vi "Demapper.vi"(8 "OFDM symbol index":u16, 9 "configuration":T4={"primary channel selector"=0.0, "last OFDM symbol index"=0, "switch format detection states"=TRUE, "format"=enum."NON_HT_OFDM", "bandwidth"=enum."20MHz"}, 10 "input valid":bool=TRUE, 11 "subcarrier channels":T1) -> (0 "subcarrier index":fxp<+/-,9,9>, 1 "subcarrier timing":T3={"subcarrier index"=0, "OFDM symbol index"=0, "frequency offset index"=0.0, "OFDM symbol start"=TRUE, "valid"=TRUE}, 2 "field map":T2, 3 "subcarrier channels out":T1)   [LabVIEW 2020]
uses:
  FPGA Bitfiles/Configuration Control.ctl
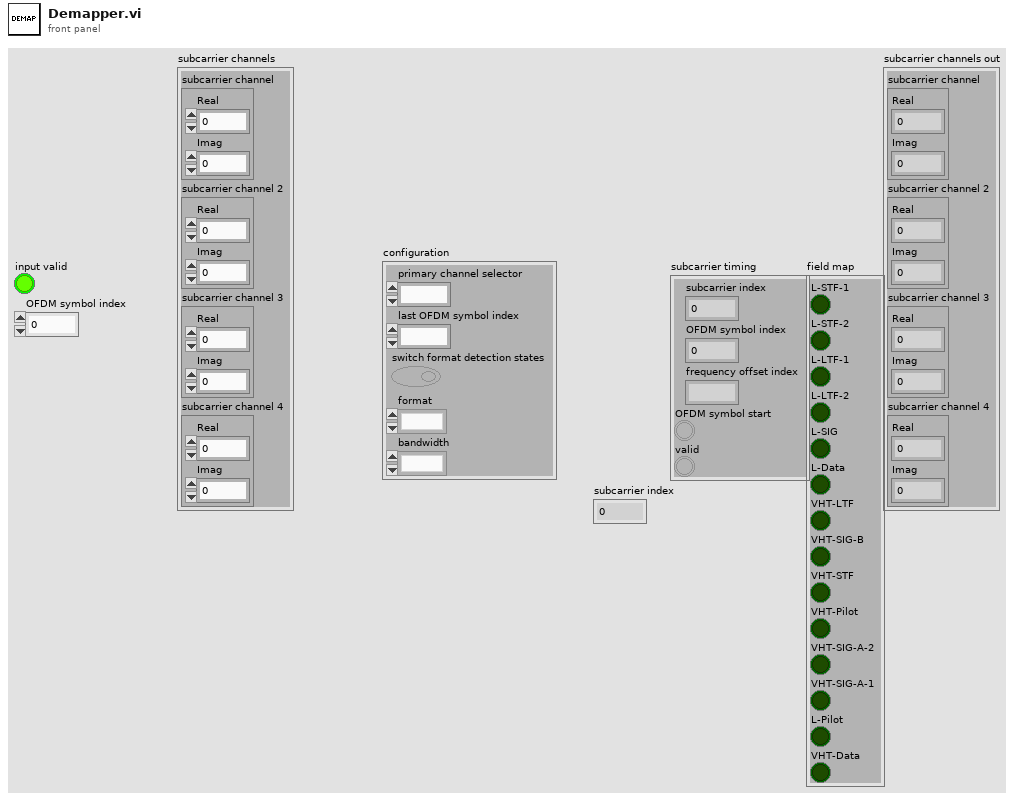
[diagram p1: front panel]
types:
  T1 = cluster{"subcarrier channel":cluster{"Real":fxp<+/-,25,4>, "Imag":fxp<+/-,25,4>}, "subcarrier channel 2":cluster{"Real":fxp<+/-,25,4>, "Imag":fxp<+/-,25,4>}, "subcarrier channel 3":cluster{"Real":fxp<+/-,25,4>, "Imag":fxp<+/-,25,4>}, "subcarrier channel 4":cluster{"Real":fxp<+/-,25,4>, "Imag":fxp<+/-,25,4>}}
  T2 = cluster{"L-STF-1":bool, "L-STF-2":bool, "L-LTF-1":bool, "L-LTF-2":bool, "L-SIG":bool, "L-Data":bool, "VHT-LTF":bool, "VHT-SIG-B":bool, "VHT-STF":bool, "VHT-Pilot":bool, "VHT-SIG-A-2":bool, "VHT-SIG-A-1":bool, "L-Pilot":bool, "VHT-Data":bool}
  T3 = cluster{"subcarrier index":u8, "OFDM symbol index":u16, "frequency offset index":fxp<+/-,9,9>, "OFDM symbol start":bool, "valid":bool}
  T4 = typedef "Configuration Control.ctl" = cluster{"primary channel selector":fxp<+,2,0>, "last OFDM symbol index":u16, "switch format detection states":bool, "format":enum16{"NON_HT_OFDM", "VHT", "NON_HT_DUP_OFDM"}, "bandwidth":enum16{"20MHz", "40MHz", "80MHz"}}
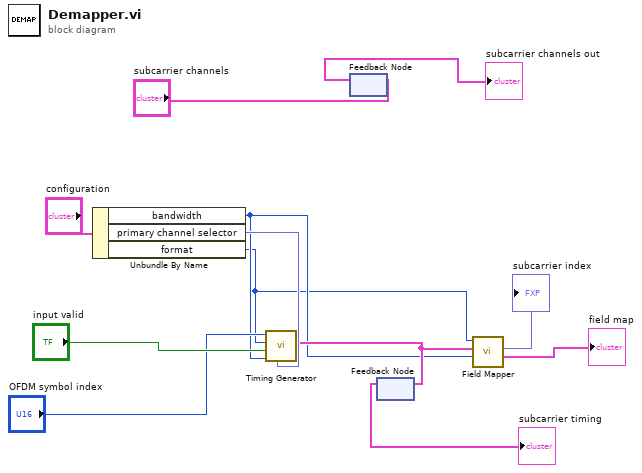
[diagram p0: block diagram]
diagram:
  n1 = Unbundle By Name("configuration") -> ("bandwidth"=w6:enum16{"20MHz", "40MHz", "80MHz"}, "primary channel selector"=w9:fxp<+,2,0>, "format"=w5:enum16{"NON_HT_OFDM", "VHT", "NON_HT_DUP_OFDM"})
  n2 = call "Timing Generator.vi"("primary channel selector"=w9, "bandwidth"=w6, "enable subcarrier counter"="input valid", "format"=w5, "OFDM symbol index"="OFDM symbol index") -> ("Cluster timing"=w7:T3)  [unwired: 6 in]
  n3 = feedback #1() -> (→"subcarrier channels out":T1)  [unwired: 1 in]
  n4 = feedback-in #1("subcarrier channels") -> ()
  n5 = feedback #2() -> (→"subcarrier timing":T3)  [unwired: 1 in]
  n6 = feedback-in #2(w7) -> ()
  n7 = call "Field Mapper.vi"("bandwidth"=w6, "subcarrier timing"=w7, "format"=w5) -> ("field map"=→"field map":T2, "subcarrier index"=→"subcarrier index":fxp<+/-,9,9>)  [unwired: 7 in]
